vi "Error 5001.vi"(8 "error in (no error)":errorcluster, 10 "Server Class Path":string) -> (0 "error out":errorcluster)   [LabVIEW 2019, in "gRPC Scripting Tools.lvlib"]
uses:
  gRPC Scripting Tools.lvlib
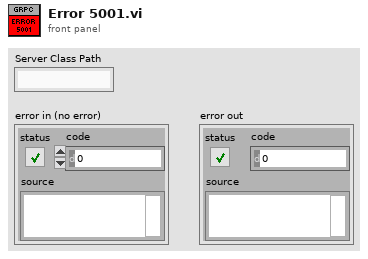
[diagram p1: front panel]
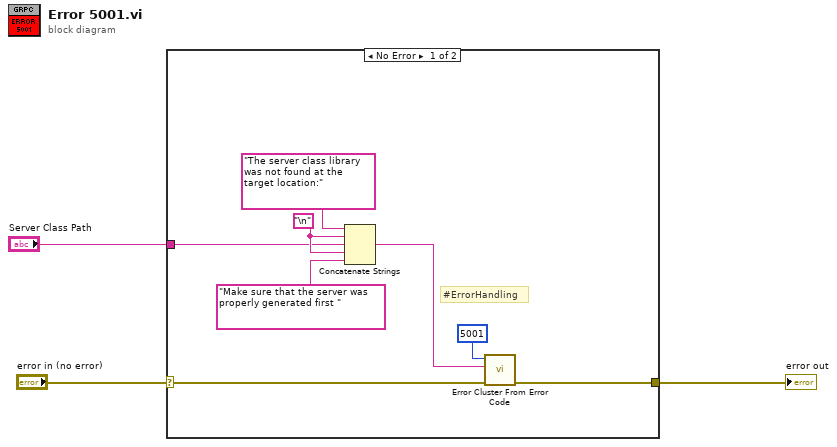
[diagram p0: block diagram]
diagram:
  n1 = case shown="No Error" "error in (no error)" {
    selector: "error in (no error)" -> [w4 w12]
    tunnel: "Server Class Path" -> [w9 _]
    tunnel: [w5 w12] -> w2
    frame No Error {
      w10 = "\n"
      # "#ErrorHandling"
      n2 = Concatenate Strings("The server class library was not found at the target location:" ("error message (\"\")"), w10, w9, w10, "Make sure that the server was properly generated first " ("string")) -> (w8:string)
      n3 = call <vilib>:"Error Cluster From Error Code.vi"("error in (no error)"=w4, "error message (\"\")"=w8, "error code (0)"=5001) -> ("error out"=w5:errorcluster)  [unwired: 6 in]
    }
    frame Error {
    }
  }
  "error out" <- w2
